vi "create array.vi"() -> ()   [LabVIEW 2018]
doc: "create array: This example is an example of creating an array."
uses:
  vi.lib/VIRobotics/opencv_yiku/Mat/Create_Mat_32F.vi
  vi.lib/VIRobotics/opencv_yiku/Mat/Mat_32F/set_2d_data.vi
  vi.lib/VIRobotics/opencv_yiku/Mat/Mat_32F/Mat_32F.lvclass
panel:
  out "2d_data":sgl[][](array[numeric])
  # "Overview: Demonstrates how to create an array.\nRequirements: Windows.\nInstructions: \n1. Run the VI."
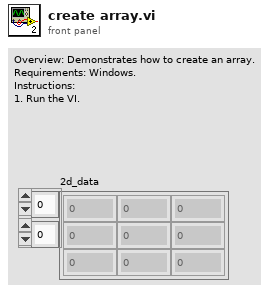
[diagram p1: front panel]
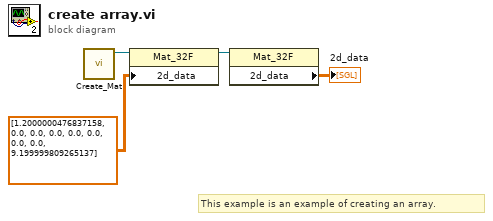
[diagram p0: block diagram]
diagram:
  # "This example is an example of creating an array."
  n1 = call-poly "Create_Mat.vi"() -> ("Mat_32F_out"=w3:refnum<class "Mat_32F.lvclass">)  [unwired: 10 in, 1 out]
  n2 = property class="Mat_32F"(reference=w3, "2d_data"=sgl[][] [[1.2, 0.0, 0.0], [0.0, 0.0, 0.0], [0.0, 0.0, 9.2]] ("Array")) -> (reference out=w2:refnum<class "Mat_32F.lvclass">)  [unwired: 1 in, 1 out]
  n3 = property class="Mat_32F"(reference=w2) -> ("2d_data"=→"2d_data":sgl[][])  [unwired: 1 in, 2 out]
